vi "Write Instrument Name to Display.vi"(8 "Error In":errorcluster, 10 "Instrument Name":string, 11 "Display Panel.lvlib:Abstract Display.lvclass":refnum<class "Abstract Display.lvclass">) -> (0 "Error Out":errorcluster, 3 "Display Panel.lvlib:Abstract Display.lvclass 2":refnum<class "Abstract Display.lvclass">)   [LabVIEW 2014, in "Display Panel.lvlib" / "Abstract Display.lvclass"]
uses:
  Abstract Display.lvclass
  Abstract Display.lvclass/Abstract Display.ctl
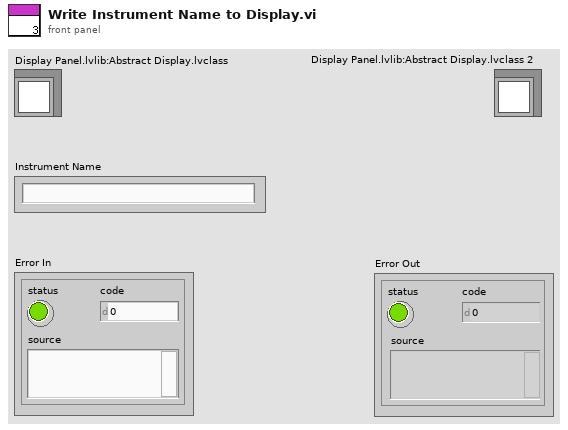
[diagram p1: front panel]
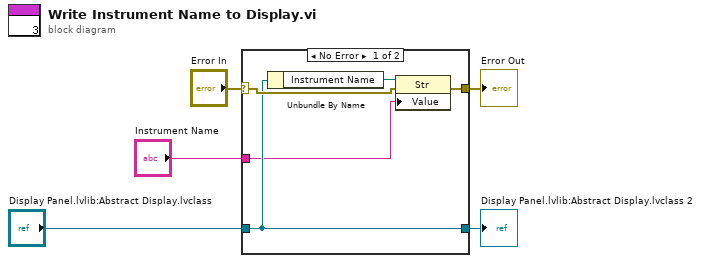
[diagram p0: block diagram]
diagram:
  n1 = case shown="No Error" "Error In" {
    selector: "Error In" -> [w9 w11]
    tunnel: [w8 w11] -> w4
    tunnel: "Display Panel.lvlib:Abstract Display.lvclass" -> [w7 w12]
    tunnel: [w7 w12] -> w2
    tunnel: "Instrument Name" -> [w6 _]
    frame No Error {
      n2 = Unbundle By Name(w7) -> ("Instrument Name"=w10:refnum<vi>)
      n3 = property class="Str"(reference=w10, error in=w9, "Value"=w6) -> (error out=w8:errorcluster)  [unwired: 1 out]
    }
    frame Error {
    }
  }
  "Error Out" <- w4
  "Display Panel.lvlib:Abstract Display.lvclass 2" <- w2
